vi "FGV_LightCommunication.vi"(7 "通訊_action":T1, 8 "error in (no error)":errorcluster, 9 "亮度":u8, 10 "通道":u8=1 min=1 max=4, 11 "VISA resource name":refnum<visa-resource-name>) -> (0 "error out":errorcluster, 3 "回應值":string)   [LabVIEW 2015]
uses:
  <userlib>/FGV/control/Control_LightCommunicationAction.ctl
  <vilib>/Instr/_visa.llb/VISA Configure Serial Port (Instr).vi
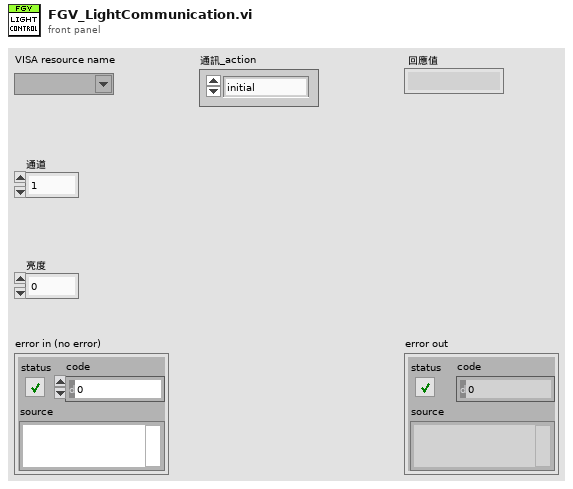
[diagram p1: front panel]
types:
  T1 = typedef "Control_LightCommunicationAction.ctl" = enum16{"initial", "開啟光源", "關閉光源", "close"}
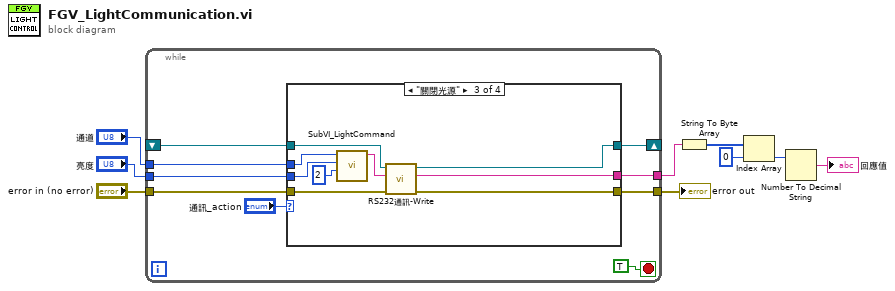
[diagram p0: block diagram]
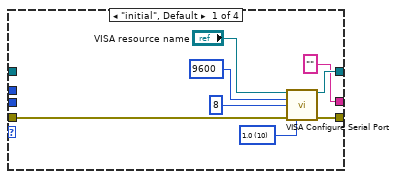
[diagram p2: hidden frame]
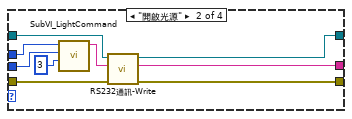
[diagram p3: hidden frame]
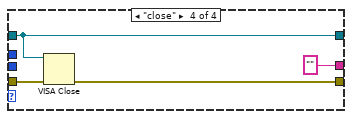
[diagram p4: hidden frame]
diagram:
  n1 = while {
    shift-right: [w14] -> _
    shift-left: _ -> [w13]
    tunnel: "error in (no error)" -> [w16]
    tunnel: [w15] -> w8
    tunnel: "亮度" -> [w12]
    tunnel: [w11] -> w2
    tunnel: "通道" -> [w10]
    stop <- TRUE stop-if-true
    n2 = case shown="\"關閉光源\"" "通訊_action" {
      tunnel: w16 -> [w26 w35 w42 w48]
      tunnel: [w25 w34 w41 w47] -> w15
      tunnel: [w24 w33 w40 w46] -> w14
      tunnel: w13 -> [_ w32 w39 w46]
      tunnel: w12 -> [_ w29 w37 _]
      tunnel: ["" ("read buffer") w28 w38 "" ("read buffer")] -> w11
      tunnel: w10 -> [_ w27 w36 _]
      frame "initial", Default {
        w19 = u16 10 items=["1.0"=10, "1.5"=15, "2.0"=20] ("stop bits (10: 1 bit)")
        n3 = call-poly "VISA Configure Serial Port"("VISA resource name"="VISA resource name", "baud rate (9600)"=u32 9600, "data bits (8)"=u16 8, "error in (no error)"=w26, "stop bits (10: 1 bit)"=w19) -> ("VISA resource name out"=w24:refnum<visa-resource-name>, "error out"=w25:errorcluster)  [unwired: 9 in]
      }
      frame "開啟光源" {
        n4 = call <userlib>:"SubVI_LightCommand.vi"("命令值"=u8 3, "亮度"=w29, "通道"=w27) -> ("concatenated string"=w31:string)  [unwired: 8 in]
        n5 = call "RS232通訊-Write.vi"("error in (no error)"=w35, "string"=w31, "VISA Refnum in"=w32) -> ("error out"=w34:errorcluster, "read buffer"=w28:string, "VISA resource name out"=w33:refnum<visa-resource-name>)  [unwired: 6 in]
      }
      frame "關閉光源" {
        n6 = call <userlib>:"SubVI_LightCommand.vi"("命令值"=u8 2, "亮度"=w37, "通道"=w36) -> ("concatenated string"=w44:string)  [unwired: 8 in]
        n7 = call "RS232通訊-Write.vi"("error in (no error)"=w42, "string"=w44, "VISA Refnum in"=w39) -> ("error out"=w41:errorcluster, "read buffer"=w38:string, "VISA resource name out"=w40:refnum<visa-resource-name>)  [unwired: 6 in]
      }
      frame "close" {
        n8 = VISA Close(VISA resource name=w46, error in (no error)=w48) -> (error out=w47:errorcluster)
      }
    }
  }
  "error out" <- w8
  n9 = String To Byte Array(string=w2) -> (unsigned byte array=w5:u8[])
  n10 = Index Array(array=w5, index=0) -> (element=w3:u8)
  n11 = Number To Decimal String(number=w3) -> (decimal integer string=→"回應值":string)  [unwired: 1 in]
